vi "STAT2 Driller Decode Data .vi"(1 "Received":bool, 7 "Driller system stat2":T1 {"Tension Sub 2"."sys register" format="%04x"; "Tension Sub 1"."sys register" format="%04x"; "PSU"."sys register" format="%04x"; "solonoid"."valve status" format="%02x"; "solonoid"."sys register" format="%04x"; "pressure 2"."sys register" format="%04x"; "pressure 1"."sys register" format="%04x"; "Controller local"."High G monitoring" format="%02x"; "Controller local"."NA" format="%02x"; "Controller local"."GPIO values" format="%02x"; "Controller local"."Relay status" format="%02x"; "Controller local"."sys register" format="%04x"}) -> (4 "Tool analog value out":dbl[](array[numeric]), 6 "Tool analog index out":u16[](array[numeric]), 8 "Tool digital value out":T7[](array[typedef]), 10 "Tool digital indexes out":u16[](array[numeric]))   [LabVIEW 2011]
uses:
  Measurments Handling/Status Digitalish.ctl
  Stroker/Stat def/Stroker system stat2.ctl
  LEINmaster/Nodes/Controller local stat2.ctl
  LEINmaster/Nodes/pressure stat2.ctl
  LEINmaster/Nodes/solonoid stat2.ctl
  LEINmaster/Nodes/PSU stat2.ctl
  LEINmaster/Nodes/tensionsub stat2.ctl
  High Level/Variable List Driller Analog.ctl
  High Level/Variable List Driller Digital.ctl
panel:
  out "error out 2":errorcluster
  in  "error in (no error)":errorcluster
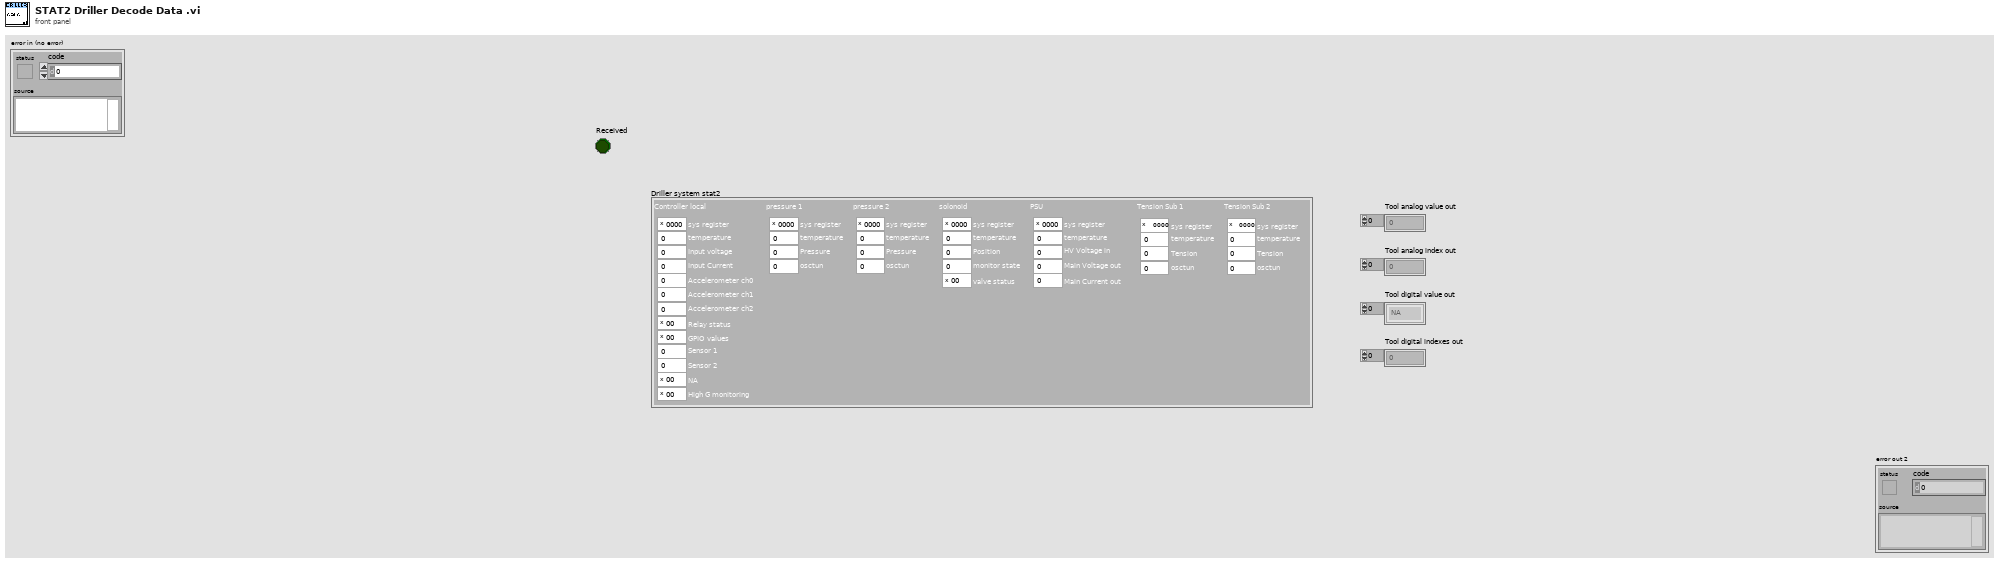
[diagram p1: front panel]
types:
  T1 = typedef "Stroker system stat2.ctl" = cluster{"Controller local":T2, "pressure 1":T3, "pressure 2":T3, "solonoid":T4, "PSU":T5, "Tension Sub 1":T6, "Tension Sub 2":T6}
  T2 = typedef "Controller local stat2.ctl" = cluster{"sys register":u16, "temperature":u16, "Input voltage":u16, "Input Current":u16, "Accelerometer ch0":u16, "Accelerometer ch1":u16, "Accelerometer ch2":u16, "Relay status":u8, "GPIO values":u8, "Sensor 1":i32, "Sensor 2":i32, "NA":u8, "High G monitoring":u8}
  T3 = typedef "pressure stat2.ctl" = cluster{"sys register":u16, "temperature":u16, "Pressure":u16, "osctun":u8}
  T4 = typedef "solonoid stat2.ctl" = cluster{"sys register":u16, "temperature":u16, "Position":i16, "monitor state":u8, "valve status":u8}
  T5 = typedef "PSU stat2.ctl" = cluster{"sys register":u16, "temperature":u16, "HV Voltage in":u16, "Main Voltage out":u16, "Main Current out":u16}
  T6 = typedef "tensionsub stat2.ctl" = cluster{"sys register":u16, "temperature":u16, "Tension":i16, "osctun":u8}
  T7 = typedef "Status Digitalish.ctl" = enum16{"NA", "False", "True"}
  T8 = typedef "Variable List Driller Analog.ctl" = enum16{"Tool max Temperature", "Tool (Solenoid) Temperature", "Tool supply Voltage", "Tool (Controller) Current", "Tool Acceleration X", "Tool Acceleration Y", "Tool Acceleration Z", "Tool (Controller) Temperature", "Tool Acceleration Sum", "Tool Inclination", "Tool Rotation", "Tool GP Sensor 1", "Tool GP Sensor 2", "Tool (Pressure 1) Temperature", "Tool Pressure 1", "Tool (Pressure 2) Temperature", "Tool Pressure 2", "Tool Motor Voltage", "Tool Motor Current", "Tool Motor Torque", "Tool Temperature sensor", "Tool weight on bit", "Tool Motor RPM", "PSU Temp", "PSU HV Voltage in", "PSU Main Voltage out", "PSU Main Current out"}
  T9 = typedef "Variable List Driller Digital.ctl" = enum16{"Tool Relay 1", "Tool Relay 2", "Tool node pressure 1", "Tool node pressure 2", "Tool node solenoid", "Tool node motor", "Tool High G Monitoring", "Tool High G Recording", "Tool High G Data ready", "Tool error Controller", "Tool error Pressure 1", "Tool error Pressure 2", "Tool error Solenoid", "Tool stopped Controller", "Tool stopped Pressure 1", "Tool stopped Pressure 2", "Tool stopped Solenoid", "Stroke Moving Out", "Stroke Moving Inn", "Oil filling mode", "Mill Bit Direction", "Reserved", "Tool Solenoid 1", "Tool Solenoid 2", "Tool Solenoid 3", "Position control", "Anchor"}
  T10 = typedef "Stat2 system error.ctl" = cluster{"Error":bool, "Has had error":bool, "Com. issue":bool}
  T11 = typedef "Stat2 system task info.ctl" = cluster{"Task":bool, "Task error":bool, "Task cnt.":u8, "Job 0":bool, "User":bool}
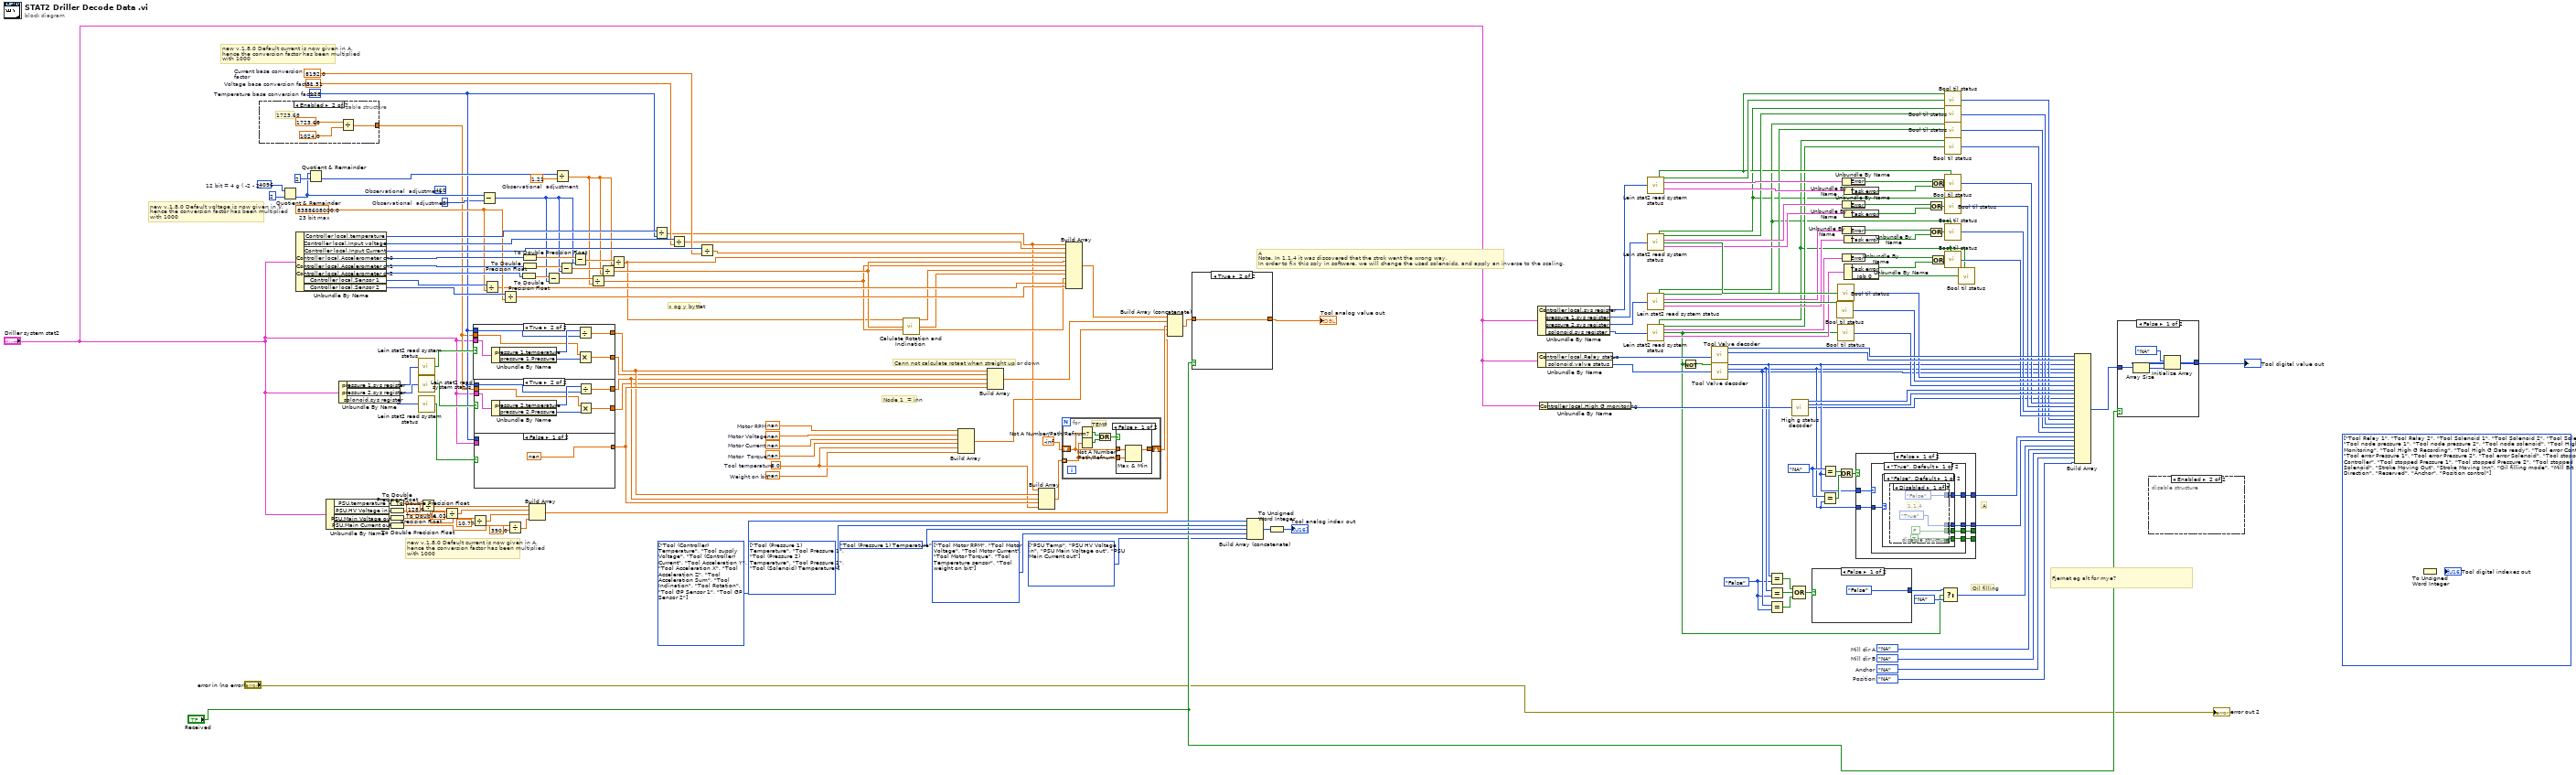
[diagram p0: block diagram]
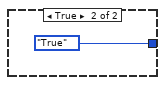
[diagram p2: hidden frame]
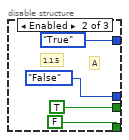
[diagram p5: hidden frame]
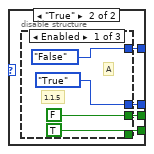
[diagram p7: hidden frame]
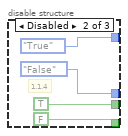
[diagram p8: hidden frame]
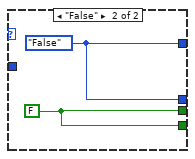
[diagram p10: hidden frame]
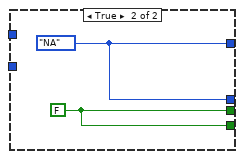
[diagram p11: hidden frame]
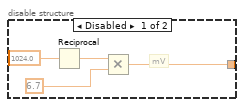
[diagram p13: hidden frame]
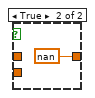
[diagram p14: hidden frame]
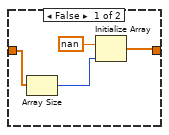
[diagram p15: hidden frame]
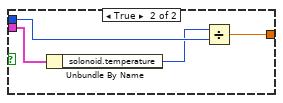
[diagram p16: hidden frame]
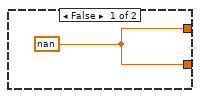
[diagram p17: hidden frame]
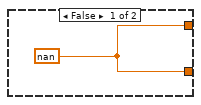
[diagram p18: hidden frame]
diagram:
  w20 = T8[] [enum."PSU Temp", enum."PSU HV Voltage in", enum."PSU Main Voltage out", enum."PSU Main Current out"] items=["Tool max Temperature", "Tool (Solenoid) Temperature", "Tool supply Voltage", "Tool (Controller) Current", "Tool Acceleration X", "Tool Acceleration Y", "Tool Acceleration Z", "Tool (Controller) Temperature", "Tool Acceleration Sum", "Tool Inclination", "Tool Rotation", "Tool GP Sensor 1", "Tool GP Sensor 2", "Tool (Pressure 1) Temperature", "Tool Pressure 1", "Tool (Pressure 2) Temperature", "Tool Pressure 2", "Tool Motor Voltage", "Tool Motor Current", "Tool Motor Torque", "Tool Temperature sensor", "Tool weight on bit", "Tool Motor RPM", "PSU Temp", "PSU HV Voltage in", "PSU Main Voltage out", "PSU Main Current out"]
  w22 = Status_Digitalish."NA"  # Position
  w23 = Status_Digitalish."NA"  # Anchor
  w24 = Status_Digitalish."NA"  # Mill dir B
  w25 = Status_Digitalish."NA"  # Mill dir A
  w33 = Status_Digitalish."False" ("x")
  w47 = Status_Digitalish."NA" ("x")
  w90 = T9[] [enum."Tool Relay 1", enum."Tool Relay 2", enum."Tool Solenoid 1", enum."Tool Solenoid 2", enum."Tool Solenoid 3", enum."Tool node pressure 1", enum."Tool node pressure 2", enum."Tool node solenoid", enum."Tool High G Monitoring", enum."Tool High G Recording", enum."Tool High G Data ready", enum."Tool error Controller", enum."Tool error Pressure 1", enum."Tool error Pressure 2", enum."Tool error Solenoid", enum."Tool stopped Controller", enum."Tool stopped Pressure 1", enum."Tool stopped Pressure 2", enum."Tool stopped Solenoid", enum."Stroke Moving Out", enum."Stroke Moving Inn", enum."Oil filling mode", enum."Mill Bit Direction", enum."Reserved", enum."Anchor", enum."Position control"] items=["Tool Relay 1", "Tool Relay 2", "Tool node pressure 1", "Tool node pressure 2", "Tool node solenoid", "Tool node motor", "Tool High G Monitoring", "Tool High G Recording", "Tool High G Data ready", "Tool error Controller", "Tool error Pressure 1", "Tool error Pressure 2", "Tool error Solenoid", "Tool stopped Controller", "Tool stopped Pressure 1", "Tool stopped Pressure 2", "Tool stopped Solenoid", "Stroke Moving Out", "Stroke Moving Inn", "Oil filling mode", "Mill Bit Direction", "Reserved", "Tool Solenoid 1", "Tool Solenoid 2", "Tool Solenoid 3", "Position control", "Anchor"]
  w103 = nan  # Weight on bit
  w104 = 0.0  # Tool temperature
  w105 = nan  # Motor  Torque
  w106 = nan  # Motor Current
  w107 = nan  # Motor Voltage
  w109 = nan  # Motor RPM
  w110 = T8[] [enum."Tool Motor RPM", enum."Tool Motor Voltage", enum."Tool Motor Current", enum."Tool Motor Torque", enum."Tool Temperature sensor", enum."Tool weight on bit"] items=["Tool max Temperature", "Tool (Solenoid) Temperature", "Tool supply Voltage", "Tool (Controller) Current", "Tool Acceleration X", "Tool Acceleration Y", "Tool Acceleration Z", "Tool (Controller) Temperature", "Tool Acceleration Sum", "Tool Inclination", "Tool Rotation", "Tool GP Sensor 1", "Tool GP Sensor 2", "Tool (Pressure 1) Temperature", "Tool Pressure 1", "Tool (Pressure 2) Temperature", "Tool Pressure 2", "Tool Motor Voltage", "Tool Motor Current", "Tool Motor Torque", "Tool Temperature sensor", "Tool weight on bit", "Tool Motor RPM", "PSU Temp", "PSU HV Voltage in", "PSU Main Voltage out", "PSU Main Current out"]
  (unwired) 410  # Observational  adjustment
  w116 = 1.21  # Observational  adjustment
  w132 = 0  # Observational  adjustment
  w136 = T8[] [enum."Tool (Pressure 1) Temperature", enum."Tool Pressure 1", enum."Tool (Pressure 2) Temperature", enum."Tool Pressure 2", enum."Tool (Solenoid) Temperature"] items=["Tool max Temperature", "Tool (Solenoid) Temperature", "Tool supply Voltage", "Tool (Controller) Current", "Tool Acceleration X", "Tool Acceleration Y", "Tool Acceleration Z", "Tool (Controller) Temperature", "Tool Acceleration Sum", "Tool Inclination", "Tool Rotation", "Tool GP Sensor 1", "Tool GP Sensor 2", "Tool (Pressure 1) Temperature", "Tool Pressure 1", "Tool (Pressure 2) Temperature", "Tool Pressure 2", "Tool Motor Voltage", "Tool Motor Current", "Tool Motor Torque", "Tool Temperature sensor", "Tool weight on bit", "Tool Motor RPM", "PSU Temp", "PSU HV Voltage in", "PSU Main Voltage out", "PSU Main Current out"]
  w148 = 8388608000.0  # 23 bit max
  w164 = 4096  # 12 bit = 4 g ( -2 - 2)
  w165 = 8192.0  # Current base conversion factor
  w167 = 31.51  # Voltage base conversion factor
  w144 = u16 128  # Temperature base conversion factor
  w137 = T8[] [enum."Tool (Controller) Temperature", enum."Tool supply Voltage", enum."Tool (Controller) Current", enum."Tool Acceleration Y", enum."Tool Acceleration X", enum."Tool Acceleration Z", enum."Tool Acceleration Sum", enum."Tool Inclination", enum."Tool Rotation", enum."Tool GP Sensor 1", enum."Tool GP Sensor 2"] items=["Tool max Temperature", "Tool (Solenoid) Temperature", "Tool supply Voltage", "Tool (Controller) Current", "Tool Acceleration X", "Tool Acceleration Y", "Tool Acceleration Z", "Tool (Controller) Temperature", "Tool Acceleration Sum", "Tool Inclination", "Tool Rotation", "Tool GP Sensor 1", "Tool GP Sensor 2", "Tool (Pressure 1) Temperature", "Tool Pressure 1", "Tool (Pressure 2) Temperature", "Tool Pressure 2", "Tool Motor Voltage", "Tool Motor Current", "Tool Motor Torque", "Tool Temperature sensor", "Tool weight on bit", "Tool Motor RPM", "PSU Temp", "PSU HV Voltage in", "PSU Main Voltage out", "PSU Main Current out"]
  # "new v.1.8.0 Default voltage is now given in V, \nhence the conversion factor has been multiplied\nwith 1000"
  # "new v.1.8.0 Default current is now given in A, \nhence the conversion factor has been multiplied\nwith 1000"
  # "new v.1.8.0 Default current is now given in A, \nhence the conversion factor has been multiplied\nwith 1000"
  # "Fjernet eg alt for mye?"
  # "Oil filling"
  # "A"
  # "A\nNote. In 1.1.4 it was discovered that the strok went the wrong way,\nIn order to fix this soly in software, we will change the used solenoids, and apply an inverse to the scaling."
  # "Node 1  = inn"
  # "Cann not calculate rotaat when streight up or down"
  # "x og y byttet"
  n1 = disable-structure shown="Enabled" {
    disable-tunnel: [w173 w177] -> w124
    frame Disabled {
      # "mV"
      n2 = Reciprocal(x=1024.0) -> (1/x=w175:dbl)
      n3 = Multiply(x=w175, y=6.7) -> (x*y=w173:dbl)
    }
    frame Enabled {
      # "1723.68"
      n4 = Divide(x=1723.68, y=1024.0 ("x")) -> (x/y=w177:dbl)
    }
  }
  n5 = Quotient & Remainder(x=w164, y=2) -> (floor(x/y)=w156:i32)  [unwired: 1 out]
  n6 = Unbundle By Name("Driller system stat2") -> ("Controller local.temperature"=w169:u16, "Controller local.Input voltage"=w168:u16, "Controller local.Input Current"=w166:u16, "Controller local.Accelerometer ch0"=w161:u16, "Controller local.Accelerometer ch1"=w159:u16, "Controller local.Accelerometer ch2"=w151:u16, "Controller local.Sensor 1"=w150:i32, "Controller local.Sensor 2"=w149:i32)
  n7 = Quotient & Remainder(x=w156, y=2) -> (floor(x/y)=w152:i32)  [unwired: 1 out]
  n8 = Unbundle By Name("Driller system stat2") -> ("PSU.temperature"=w19:u16, "PSU.HV Voltage in"=w17:u16, "PSU.Main Voltage out"=w16:u16, "PSU.Main Current out"=w18:u16)
  n9 = Unbundle By Name("Driller system stat2") -> ("pressure 1.sys register"=w170:u16, "pressure 2.sys register"=w172:u16, "solonoid.sys register"=w171:u16)
  n10 = To Double Precision Float(number=w19) -> (double precision float=w15:dbl)
  n11 = To Double Precision Float(number=w17) -> (double precision float=w9:dbl)
  n12 = To Double Precision Float(number=w16) -> (double precision float=w11:dbl)
  n13 = To Double Precision Float(number=w18) -> (double precision float=w4:dbl)
  n14 = call "Lein stat2 read system status.vi"("sys register"=w170) -> ("Connected"=w147:bool)  [unwired: 7 in, 7 out]
  n15 = call "Lein stat2 read system status.vi"("sys register"=w172) -> ("Connected"=w146:bool)  [unwired: 7 in, 7 out]
  n16 = call "Lein stat2 read system status.vi"("sys register"=w171) -> ("Connected"=w145:bool)  [unwired: 7 in, 7 out]
  n17 = Divide(x=w15, y=128.0) -> (x/y=w13:dbl)
  n18 = Divide(x=w9, y=1.02) -> (x/y=w8:dbl)
  n19 = Divide(x=w11, y=10.77) -> (x/y=w10:dbl)
  n20 = case shown="True" w147 {
    tunnel: w124 -> [_ w183]
    tunnel: w144 -> [_ w185]
    tunnel: "Driller system stat2" -> [_ w187]
    tunnel: [w180 w182] -> w122
    tunnel: [w180 w181] -> w115
    frame False {
      w180 = nan
    }
    frame True {
      n21 = Unbundle By Name(w187) -> ("pressure 1.temperature"=w186:u16, "pressure 1.Pressure"=w184:u16)
      n22 = Divide(x=w186, y=w185) -> (x/y=w182:dbl)
      n23 = Multiply(x=w183, y=w184) -> (x*y=w181:dbl)
    }
  }
  n24 = case shown="True" w146 {
    tunnel: w124 -> [_ w191]
    tunnel: w144 -> [_ w193]
    tunnel: "Driller system stat2" -> [_ w195]
    tunnel: [w188 w190] -> w121
    tunnel: [w188 w189] -> w114
    frame False {
      w188 = nan
    }
    frame True {
      n25 = Unbundle By Name(w195) -> ("pressure 2.temperature"=w194:u16, "pressure 2.Pressure"=w192:u16)
      n26 = Divide(x=w194, y=w193) -> (x/y=w190:dbl)
      n27 = Multiply(x=w191, y=w192) -> (x*y=w189:dbl)
    }
  }
  n28 = case shown="False" w145 {
    tunnel: w144 -> [_ w199]
    tunnel: "Driller system stat2" -> [_ w200]
    tunnel: [nan w197] -> w123
    frame False {
    }
    frame True {
      n29 = Unbundle By Name(w200) -> ("solonoid.temperature"=w198:u16)
      n30 = Divide(x=w198, y=w199) -> (x/y=w197:dbl)
    }
  }
  n31 = Subtract(x=w156, y=w132) -> (x-y=w133:i32)
  n32 = Divide(x=w150, y=w148) -> (x/y=w140:dbl)
  n33 = Divide(x=w149, y=w148) -> (x/y=w141:dbl)
  n34 = Divide(x=w4, y=390.0) -> (x/y=w5:dbl)
  n35 = To Double Precision Float(number=w151) -> (double precision float=w158:dbl)
  n36 = To Double Precision Float(number=w161) -> (double precision float=w162:dbl)
  n37 = To Double Precision Float(number=w159) -> (double precision float=w160:dbl)
  n38 = Build Array(w13, w8, w10, w5) -> (w2:dbl[])
  n39 = Subtract(x=w158, y=w133) -> (x-y=w153:dbl)
  n40 = Divide(x=w152, y=w116) -> (x/y=w131:dbl)
  n41 = Subtract(x=w160, y=w133) -> (x-y=w154:dbl)
  n42 = Subtract(x=w162, y=w133) -> (x-y=w155:dbl)
  n43 = Divide(x=w153, y=w131) -> (x/y=w129:dbl)
  n44 = Divide(x=w154, y=w131) -> (x/y=w130:dbl)
  n45 = Divide(x=w155, y=w131) -> (x/y=w128:dbl)
  n46 = Divide(x=w169, y=w144) -> (x/y=w120:dbl)
  n47 = Divide(x=w168, y=w167) -> (x/y=w143:dbl)
  n48 = Divide(x=w166, y=w165) -> (x/y=w142:dbl)
  n49 = call "Calulate Rotation and Inclination.vi"("Ch 0"=w128, "Ch 1"=w130, "Ch 2"=w129) -> ("Magnitude XYZ(g)"=w126:dbl, "Inclination"=w125:dbl, "Rotation"=w127:dbl)  [unwired: 10 in]
  n50 = Build Array(w109, w107, w106, w105, w104, w103) -> (w108:dbl[])
  n51 = Build Array(w122, w115, w121, w114, w123) -> (w138:dbl[])
  n52 = Build Array(w120, w122, w121, w123, w104) -> (w119:dbl[])
  n53 = for {
    tunnel: w119 -> [w204] mode=indexing
    shift-right: [w206] -> w117
    shift-left: -inf -> [w205]
    # "TEMP"
    n54 = Not A Number/Path/Refnum?(number/path/refnum=w205) -> (NaN/Path/Refnum?=w202:bool)
    n55 = Not A Number/Path/Refnum?(number/path/refnum=w204) -> (NaN/Path/Refnum?=w203:bool)
    n56 = Or(x=w202, y=w203) -> (x .or. y?=w201:bool)
    n57 = case shown="False" w201 {
      tunnel: [w209 nan] -> w206
      tunnel: w205 -> [w208 _]
      tunnel: w204 -> [w207 _]
      frame False {
        n58 = Max & Min(x=w208, y=w207) -> (max(x,y)=w209:dbl)  [unwired: 1 out]
      }
      frame True {
      }
    }
  }
  n59 = Build Array(w120, w143, w142, w128, w130, w129, w126, w125, w127, w140, w141) -> (w139:dbl[])
  n60 = Build Array (concatenate)(w139, w138, w117, w108, w2) -> (w134:dbl[])
  n61 = case shown="True" "Received" {
    tunnel: [w211 w215] -> w113
    tunnel: w134 -> [w214 w215]
    frame False {
      n62 = Array Size(array=w214) -> (size(s)=w213:i32)
      n63 = Initialize Array(nan ("element"), w213) -> (w211:dbl[])
    }
    frame True {
    }
  }
  "Tool analog value out" <- w113
  n64 = Build Array (concatenate)(w137, w136, Variable_List_Driller_Analog."Tool (Pressure 1) Temperature" ("Action"), w110, w20) -> (w135:T8[])
  n65 = To Unsigned Word Integer(number=w135) -> (unsigned 16bit integer=→"Tool analog index out":u16[])
  n66 = Unbundle By Name("Driller system stat2") -> ("Controller local.sys register"=w80:u16, "pressure 1.sys register"=w98:u16, "pressure 2.sys register"=w96:u16, "solonoid.sys register"=w97:u16)
  n67 = Unbundle By Name("Driller system stat2") -> ("Controller local.Relay status"=w102:u8, "solonoid.valve status"=w101:u8)
  n68 = Unbundle By Name("Driller system stat2") -> ("Controller local.High G monitoring"=w88:u8)
  n69 = call "Lein stat2 read system status.vi"("sys register"=w80) -> ("Force NA"=w53:bool, "Stopped"=w60:bool, "Error"=w79:T10, "Task"=w73:T11)  [unwired: 7 in, 4 out]
  n70 = call "Lein stat2 read system status.vi"("sys register"=w98) -> ("Force NA"=w41:bool, "Stopped"=w59:bool, "Error"=w85:T10, "Connected"=w92:bool, "Task"=w72:T11)  [unwired: 7 in, 3 out]
  n71 = call "Lein stat2 read system status.vi"("sys register"=w96) -> ("Force NA"=w42:bool, "Stopped"=w58:bool, "Error"=w84:T10, "Connected"=w94:bool, "Task"=w71:T11)  [unwired: 7 in, 3 out]
  n72 = call "Lein stat2 read system status.vi"("sys register"=w97) -> ("Force NA"=w50:bool, "Stopped"=w52:bool, "Error"=w83:T10, "Connected"=w21:bool, "Task"=w70:T11)  [unwired: 7 in, 3 out]
  n73 = Not(x=w21) -> (.not. x?=w43:bool)
  n74 = call "Tool Valve decoder.vi"("Valv Relay code"=w102) -> ("Valve LSB(0)"=w100:T7, "Valve 1"=w99:T7)  [unwired: 10 in, 3 out]
  n75 = call "Tool Valve decoder.vi"("Force NA(F)"=w43, "Valv Relay code"=w101) -> ("Valve LSB(0)"=w36:T7, "Valve 1"=w35:T7, "Valve 2"=w34:T7)  [unwired: 9 in, 2 out]
  n76 = Equal?(x=w36, y=w33) -> (x = y?=w32:bool)
  n77 = Equal?(x=w35, y=w33) -> (x = y?=w31:bool)
  n78 = Equal?(x=w34, y=w33) -> (x = y?=w30:bool)
  n79 = call "High g status decoder.vi"("High G Code"=w88) -> ("Monitoring"=w87:T7, "Recording"=w86:T7, "Data ready"=w1:T7)  [unwired: 11 in, 1 out]
  n80 = Compound Arithmetic op=OR(w32, w31, w30) -> (w29:bool)
  n81 = case shown="False" w29 {
    tunnel: [Status_Digitalish."False" ("x") Status_Digitalish."True" ("x")] -> w28
    frame False {
    }
    frame True {
    }
  }
  n82 = Equal?(x=w47, y=w35) -> (x = y?=w44:bool)
  n83 = Equal?(x=w47, y=w36) -> (x = y?=w45:bool)
  n84 = call "Bool til status.vi"("Boolean"=w94) -> ("Status"=w93:T7)  [unwired: 8 in]
  n85 = call "Bool til status.vi"("Boolean"=w92) -> ("Status"=w91:T7)  [unwired: 8 in]
  n86 = call "Bool til status.vi"("Boolean"=w21) -> ("Status"=w95:T7)  [unwired: 8 in]
  n87 = Or(x=w45, y=w44) -> (x .or. y?=w46:bool)
  n88 = Unbundle By Name(w79) -> ("Error"=w78:bool)
  n89 = Unbundle By Name(w85) -> ("Error"=w82:bool)
  n90 = Unbundle By Name(w84) -> ("Error"=w81:bool)
  n91 = Unbundle By Name(w83) -> ("Error"=w69:bool)
  n92 = Unbundle By Name(w73) -> ("Task error"=w64:bool)
  n93 = Unbundle By Name(w72) -> ("Task error"=w63:bool)
  n94 = Unbundle By Name(w71) -> ("Task error"=w62:bool)
  n95 = Unbundle By Name(w70) -> ("Task error"=w61:bool, "Job 0"=w51:bool)
  n96 = case shown="False" w46 {
    tunnel: w36 -> [w223 _]
    tunnel: [w222 w256] -> w49
    tunnel: [w221 w256] -> w48
    tunnel: w35 -> [w220 _]
    tunnel: [w219 w255] -> _
    tunnel: [w218 w255] -> _
    frame False {
      n97 = case shown="\"True\", Default" w223 {
        tunnel: [w228 w254] -> w222
        tunnel: [w227 w254] -> w221
        tunnel: w220 -> [w226 _]
        tunnel: [w225 w253] -> w219
        tunnel: [w224 w253] -> w218
        frame "True", Default {
          n98 = case shown="\"False\", Default" w226 {
            tunnel: [w232 w244] -> w228
            tunnel: [w231 w243] -> w227
            tunnel: [w229 w242] -> w225
            tunnel: [w230 w241] -> w224
            frame "False", Default {
              n99 = disable-structure shown="Disabled" {
                disable-tunnel: [Status_Digitalish."False" ("Valve LSB(0)") Status_Digitalish."True" ("Valve LSB(0)") _] -> w232
                disable-tunnel: [Status_Digitalish."True" ("Valve LSB(0)") Status_Digitalish."False" ("Valve LSB(0)") _] -> w231
                disable-tunnel: [TRUE FALSE _] -> w230
                disable-tunnel: [FALSE TRUE _] -> w229
                frame Disabled {
                  # "1.1.4"
                }
                frame Enabled {
                  # "A"
                  # "1.1.5"
                }
                frame Disabled {
                }
              }
            }
            frame "True" {
              n100 = disable-structure shown="Enabled" {
                disable-tunnel: [Status_Digitalish."False" ("Valve LSB(0)") Status_Digitalish."True" ("Valve LSB(0)") _] -> w244
                disable-tunnel: [Status_Digitalish."True" ("Valve LSB(0)") Status_Digitalish."False" ("Valve LSB(0)") _] -> w243
                disable-tunnel: [FALSE TRUE _] -> w242
                disable-tunnel: [TRUE FALSE _] -> w241
                frame Enabled {
                  # "A"
                  # "1.1.5"
                }
                frame Disabled {
                  # "1.1.4"
                }
                frame Disabled {
                }
              }
            }
          }
        }
        frame "False" {
          w253 = FALSE
          w254 = Status_Digitalish."False" ("Valve LSB(0)")
        }
      }
    }
    frame True {
      w255 = FALSE
      w256 = Status_Digitalish."NA" ("Valve LSB(0)")
    }
  }
  n101 = Or(x=w82, y=w63) -> (x .or. y?=w66:bool)
  n102 = Or(x=w81, y=w62) -> (x .or. y?=w67:bool)
  n103 = Or(x=w78, y=w64) -> (x .or. y?=w65:bool)
  n104 = Or(x=w69, y=w61) -> (x .or. y?=w68:bool)
  n105 = Select(t=w28, s=w21, f=Status_Digitalish."NA") -> (s? t:f=w26:T7)
  n106 = call "Bool til status.vi"("Force NA(F)"=w53, "Boolean"=w60) -> ("Status"=w57:T7)  [unwired: 7 in]
  n107 = call "Bool til status.vi"("Force NA(F)"=w41, "Boolean"=w59) -> ("Status"=w56:T7)  [unwired: 7 in]
  n108 = call "Bool til status.vi"("Force NA(F)"=w42, "Boolean"=w58) -> ("Status"=w55:T7)  [unwired: 7 in]
  n109 = call "Bool til status.vi"("Force NA(F)"=w50, "Boolean"=w52) -> ("Status"=w54:T7)  [unwired: 7 in]
  n110 = call "Bool til status.vi"("Force NA(F)"=w53, "Boolean"=w65) -> ("Status"=w77:T7)  [unwired: 7 in]
  n111 = call "Bool til status.vi"("Force NA(F)"=w41, "Boolean"=w66) -> ("Status"=w76:T7)  [unwired: 7 in]
  n112 = call "Bool til status.vi"("Force NA(F)"=w42, "Boolean"=w67) -> ("Status"=w75:T7)  [unwired: 7 in]
  n113 = call "Bool til status.vi"("Force NA(F)"=w50, "Boolean"=w68) -> ("Status"=w74:T7)  [unwired: 7 in]
  n114 = call "Bool til status.vi"("Force NA(F)"=w50, "Boolean"=w51) -> ()  [unwired: 7 in, 1 out]
  n115 = Build Array(w100, w99, w36, w35, w34, w91, w93, w95, w87, w86, w1, w77, w76, w75, w74, w57, w56, w55, w54, w49, w48, w26, w25, w24, w23, w22) -> (w89:T7[])
  n116 = case shown="False" "Received" {
    tunnel: [w258 w261] -> w39
    tunnel: w89 -> [w260 w261]
    frame False {
      n117 = Array Size(array=w260) -> (size(s)=w259:i32)
      n118 = Initialize Array(Status_Digitalish."NA" ("Status"), w259) -> (w258:T7[])
    }
    frame True {
    }
  }
  "Tool digital value out" <- w39
  n119 = disable-structure shown="Enabled" {
    frame Disabled {
      n120 = case shown="\"Strok out = node 1\"" {
        selector: _ -> [_ _]
        tunnel: _ -> [w263 w264]
        tunnel: _ -> [w262 w265]
        tunnel: [w263 w265] -> _
        tunnel: [w262 w264] -> _
        frame "Stroke in = node 1", Default {
        }
        frame "Strok out = node 1" {
        }
      }
    }
    frame Enabled {
    }
  }
  n121 = To Unsigned Word Integer(number=w90) -> (unsigned 16bit integer=→"Tool digital indexes out":u16[])
  "error out 2" <- "error in (no error)"
